vi "LoaderWithColor.vi"() -> ()   [LabVIEW 2019]
uses:
  <vilib>/Rock Robotics/WPI/ThirdParty/Phoenix-LabVIEW/Motor Controller/Controls/CTRE_Phoenix_MotorControl_ControlMode.ctl
  Robot Global Data.vi
  <vilib>/Rock Robotics/WPI/ThirdParty/Phoenix-LabVIEW/Motor Controller/Get/CTRE_Phoenix_MotorController_GetSelectedSensorData.vi
panel:
  out "Position":i32
  in  "counter":dbl
  in  "Output":dbl
  out "SEE?":bool
  out "intake":bool
  in  "error in":errorcluster
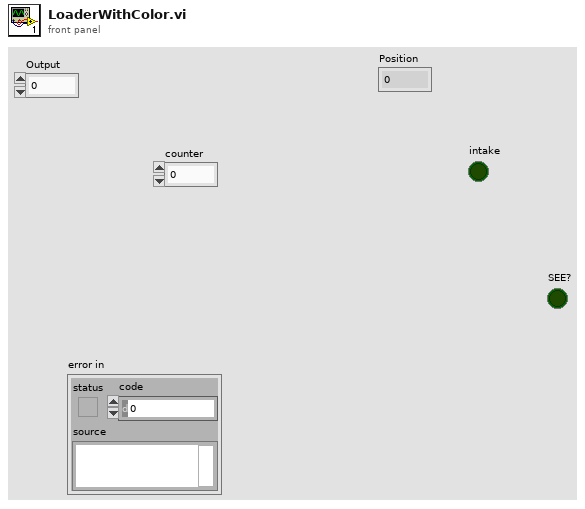
[diagram p1: front panel]
types:
  T1 = typedef "WPI_JoystickDevRef.ctl" = cluster{"Device":T2}
  T2 = typedef "WPI_JoystickDeviceEnum.ctl" = enum16{"USB 0", "USB 1", "USB 2", "USB 3", "USB 4", "USB 5"}
  T3 = typedef "WPI_MotorControlDeviceRef.ctl" = cluster{"DeviceStatus":errorcluster, "Type":T4, "PWM":cluster{"PWM Channel":T5, "DeadBand":T6}, "CAN":cluster{"Device Number":u8, "SetOutput VI Ref":variant, "GetOutput VI Ref":variant, "Enable VI Ref":variant, "Disable VI Ref":variant, "Data":variant}, "Invert":bool, "DIO PWM":cluster{"PWM \"Enable\" Channel":T5, "DIOChannel":T7, "PWM Rate":dbl}}
  T4 = typedef "WPI_MotorControlType.ctl" = enum16{"PWM", "CAN", "DIO PWM"}
  T5 = typedef "FPGA_DIOPWMChannel.ctl" = enum8{"PWM 0", "PWM 1", "PWM 2", "PWM 3", "PWM 4", "PWM 5", "PWM 6", "PWM 7", "PWM 8", "PWM 9", "PWM MXP 0", "PWM MXP 1", "PWM MXP 2", "PWM MXP 3", "PWM MXP 4", "PWM MXP 5", "PWM MXP 6", "PWM MXP 7", "PWM MXP 8", "PWM MXP 9", "Invalid"}
  T6 = typedef "WPI_PWMDeadband.ctl" = cluster{"Name":string, "maxPositivePwm":i32, "minPositivePwm":i32, "centerPwm":i32, "maxNegativePwm":i32, "minNegativePwm":i32, "angularRange":u16}
  T7 = typedef "FPGA_DIOChannel.ctl" = enum8{"DIO 0", "DIO 1", "DIO 2", "DIO 3", "DIO 4", "DIO 5", "DIO 6", "DIO 7", "DIO 8", "DIO 9", "DIO MXP 0", "DIO MXP 1", "DIO MXP 2", "DIO MXP 3", "DIO MXP 4", "DIO MXP 5", "DIO MXP 6", "DIO MXP 7", "DIO MXP 8", "DIO MXP 9", "DIO MXP 10", "DIO MXP 11", "DIO MXP 12", "DIO MXP 13", "DIO MXP 14", "DIO MXP 15", "SPI Port CS1", "SPI Port CS2", "SPI Port CS3", "SPI Port MISO", "SPI Port MOSI", "Invalid"}
  T8 = typedef "CTRE_Phoenix_MotorControl_ControlMode.ctl" = u16
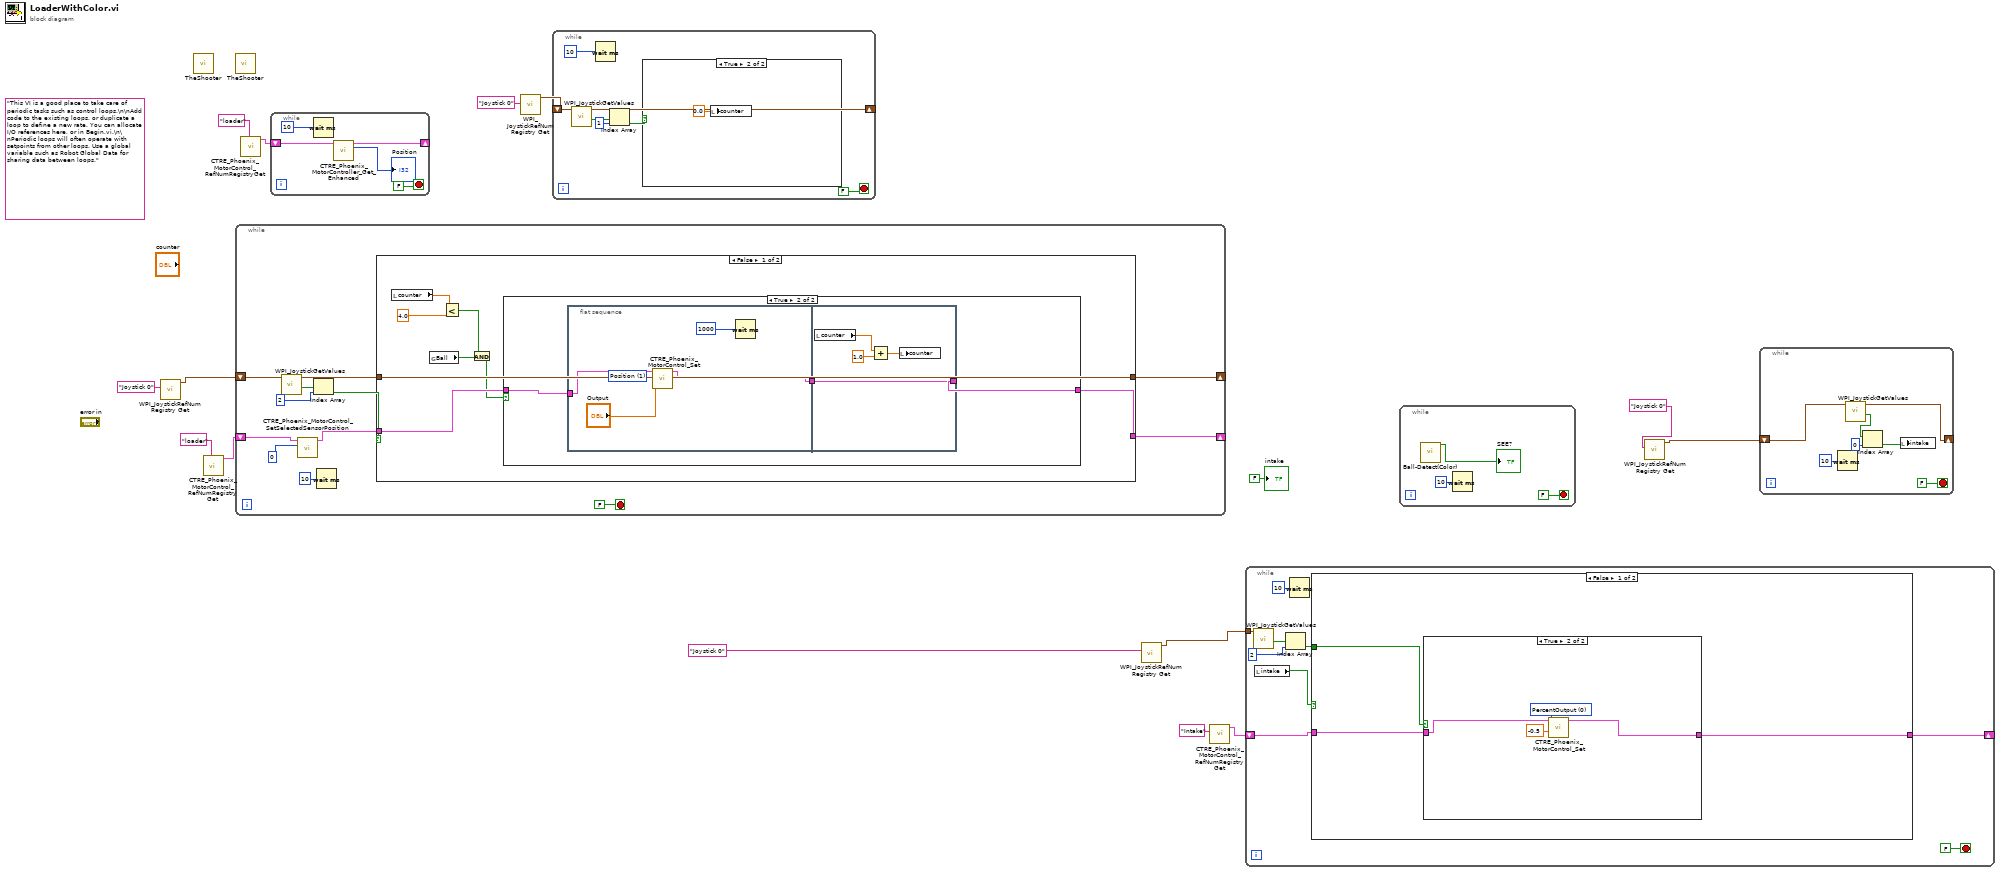
[diagram p0: block diagram]
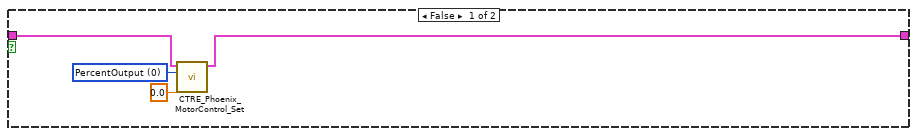
[diagram p3: hidden frame]
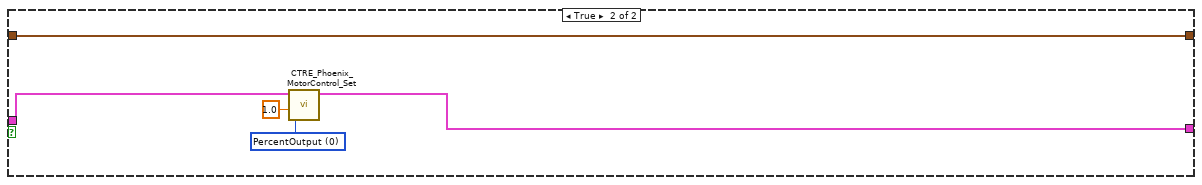
[diagram p4: hidden frame]
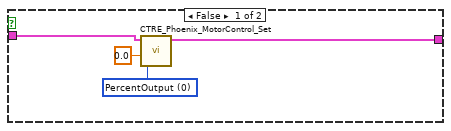
[diagram p5: hidden frame]
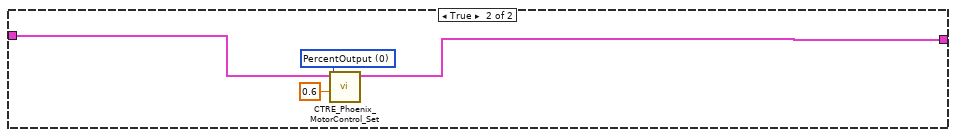
[diagram p6: hidden frame]
diagram:
  (unwired) "This VI is a good place to take care of periodic tasks such as control loops.\n\nAdd code to the existing loops, or duplicate a loop to define a new rate. You can allocate I/O references here, or in Begin.vi.\n\nPeriodic loops will often operate with setpoints from other loops. Use a global variable such as Robot Global Data for sharing data between loops."
  n1 = call <vilib>:"WPI_JoystickRefNum Registry Get.vi"("refnum name"="Joystick 0") -> ("JoystickDevRef"=w7:T1)  [unwired: 9 in, 1 out]
  n2 = call "TheShooter.vi"() -> ()  [unwired: 12 in]
  n3 = call <vilib>:"CTRE_Phoenix_MotorControl_RefNumRegistryGet.vi"("refnum name"="loader") -> ("PhoenixMotorControlDevRef"=w9:T3)  [unwired: 9 in, 1 out]
  n4 = call "TheShooter.vi"() -> ()  [unwired: 12 in]
  n5 = while {
    shift-right: [w25] -> _
    shift-left: w9 -> [w17]
    shift-right: [w21] -> _
    shift-left: w7 -> [w23]
    stop <- FALSE stop-if-true
    n6 = call <vilib>:"WPI_JoystickGetValues.vi"("JoystickDevRef"=w23) -> ("Buttons"=w24:bool[], "JoystickDevRef"=w22:T1)  [unwired: 6 in, 3 out]
    n7 = call <vilib>:"CTRE_Phoenix_MotorControl_SetSelectedSensorPosition.vi"("New Sensor Position"=0, "PhoenixMotorControlDevRef"=w17) -> ("PhoenixMotorControlDevRef"=w16:T3)  [unwired: 8 in, 1 out]
    n8 = Index Array(array=w24, index=2) -> (element=w20:bool)
    n9 = Wait (ms)(milliseconds to wait=u32 10) -> ()  [unwired: 1 out]
    n10 = case shown="False" w20 {
      tunnel: [w34 w53] -> w25
      tunnel: w16 -> [w35 w54]
      tunnel: w22 -> [w33 w52]
      tunnel: [w33 w52] -> w21
      frame False {
        n11 = local read "counter"() -> (w32:dbl)
        n12 = global read "Robot Global Data.vi" "Ball"() -> (w30:bool)
        n13 = Less?(x=w32, y=4.0) -> (x < y?=w28:bool)
        n14 = And(x=w28, y=w30) -> (x .and. y?=w29:bool)
        n15 = case shown="True" w29 {
          tunnel: w35 -> [w37 w40]
          tunnel: [w36 w42] -> w34
          frame False {
            w39 = T8 0 items=["PercentOutput"=0, "Position"=1, "Velocity"=2, "Current"=3, "Follower"=5, "MotionProfile"=6, "MotionMagic"=7, "MotionProfileArc"=10, "Disabled"=15] ("Control Mode")
            n16 = call <vilib>:"CTRE_Phoenix_MotorControl_Set.vi"("Output"=0.0, "Control Mode"=w39, "PhoenixMotorControlDevRef"=w37) -> ("PhoenixMotorControlDevRef"=w36:T3)  [unwired: 7 in, 1 out]
          }
          frame True {
            n17 = flat-sequence {
              tunnel: [w45] -> w41
              tunnel: w40 -> [w46]
              tunnel: [w51] -> w42
              tunnel: w41 -> [w51]
              frame #0 {
                w44 = T8 1 items=["PercentOutput"=0, "Position"=1, "Velocity"=2, "Current"=3, "Follower"=5, "MotionProfile"=6, "MotionMagic"=7, "MotionProfileArc"=10, "Disabled"=15] ("Control Mode")
                n18 = call <vilib>:"CTRE_Phoenix_MotorControl_Set.vi"("Output"="Output", "Control Mode"=w44, "PhoenixMotorControlDevRef"=w46) -> ("PhoenixMotorControlDevRef"=w45:T3)  [unwired: 7 in, 1 out]
                n19 = Wait (ms)(milliseconds to wait=u32 1000 ("millisecond timer value")) -> ()  [unwired: 1 out]
              }
              frame #1 {
                n20 = local read "counter"() -> (w49:dbl)
                n21 = Add(x=w49, y=1.0) -> (x+y=w50:dbl)
                n22 = local write "counter"(w50) -> ()
              }
            }
          }
        }
      }
      frame True {
        w55 = T8 0 items=["PercentOutput"=0, "Position"=1, "Velocity"=2, "Current"=3, "Follower"=5, "MotionProfile"=6, "MotionMagic"=7, "MotionProfileArc"=10, "Disabled"=15] ("Control Mode")
        n23 = call <vilib>:"CTRE_Phoenix_MotorControl_Set.vi"("Output"=1.0, "Control Mode"=w55, "PhoenixMotorControlDevRef"=w54) -> ("PhoenixMotorControlDevRef"=w53:T3)  [unwired: 7 in, 1 out]
      }
    }
  }
  n24 = call <vilib>:"CTRE_Phoenix_MotorControl_RefNumRegistryGet.vi"("refnum name"="loader") -> ("PhoenixMotorControlDevRef"=w1:T3)  [unwired: 9 in, 1 out]
  n25 = while {
    shift-right: [w60] -> _
    shift-left: w1 -> [w61]
    stop <- FALSE stop-if-true
    n26 = Wait (ms)(milliseconds to wait=u32 10 ("millisecond timer value")) -> ()  [unwired: 1 out]
    n27 = call-poly <vilib>:"CTRE_Phoenix_MotorController_Get_Enhanced.vi"("PhoenixMotorControlDevRef"=w61) -> ("PhoenixMotorControlDevRef"=w60:T3, "Position (Raw Sensor Units)"=→"Position":i32)  [unwired: 11 in, 2 out]
  }
  n28 = call <vilib>:"WPI_JoystickRefNum Registry Get.vi"("refnum name"="Joystick 0") -> ("JoystickDevRef"=w3:T1)  [unwired: 9 in, 1 out]
  n29 = while {
    shift-right: [w64] -> _
    shift-left: w3 -> [w66]
    stop <- FALSE stop-if-true
    n30 = call <vilib>:"WPI_JoystickGetValues.vi"("JoystickDevRef"=w66) -> ("Buttons"=w68:bool[], "JoystickDevRef"=w64:T1)  [unwired: 6 in, 3 out]
    n31 = Wait (ms)(milliseconds to wait=u32 10 ("millisecond timer value")) -> ()  [unwired: 1 out]
    n32 = Index Array(array=w68, index=1) -> (element=w65:bool)
    n33 = case shown="True" w65 {
      frame False {
      }
      frame True {
        n34 = local write "counter"(0.0 ("counter")) -> ()
      }
    }
  }
  n35 = call <vilib>:"WPI_JoystickRefNum Registry Get.vi"("refnum name"="Joystick 0") -> ("JoystickDevRef"=w5:T1)  [unwired: 9 in, 1 out]
  n36 = call <vilib>:"CTRE_Phoenix_MotorControl_RefNumRegistryGet.vi"("refnum name"="Intake") -> ("PhoenixMotorControlDevRef"=w12:T3)  [unwired: 9 in, 1 out]
  n37 = while {
    shift-right: [w75] -> _
    shift-left: w12 -> [w76]
    tunnel: w5 -> [w71]
    stop <- FALSE stop-if-true
    n38 = call <vilib>:"WPI_JoystickGetValues.vi"("JoystickDevRef"=w71) -> ("Buttons"=w72:bool[])  [unwired: 6 in, 4 out]
    n39 = local read "intake"() -> (w74:bool)
    n40 = Index Array(array=w72, index=2) -> (element=w70:bool)
    n41 = Wait (ms)(milliseconds to wait=u32 10) -> ()  [unwired: 1 out]
    n42 = case shown="False" w74 {
      tunnel: w76 -> [w81 w93]
      tunnel: [w80 w92] -> w75
      tunnel: w70 -> [w79 _]
      frame False {
        n43 = case shown="True" w79 {
          tunnel: w81 -> [w83 w87]
          tunnel: [w82 w86] -> w80
          frame False {
            w85 = T8 0 items=["PercentOutput"=0, "Position"=1, "Velocity"=2, "Current"=3, "Follower"=5, "MotionProfile"=6, "MotionMagic"=7, "MotionProfileArc"=10, "Disabled"=15] ("Control Mode")
            n44 = call <vilib>:"CTRE_Phoenix_MotorControl_Set.vi"("Output"=0.0, "Control Mode"=w85, "PhoenixMotorControlDevRef"=w83) -> ("PhoenixMotorControlDevRef"=w82:T3)  [unwired: 7 in, 1 out]
          }
          frame True {
            w89 = T8 0 items=["PercentOutput"=0, "Position"=1, "Velocity"=2, "Current"=3, "Follower"=5, "MotionProfile"=6, "MotionMagic"=7, "MotionProfileArc"=10, "Disabled"=15] ("Control Mode")
            n45 = call <vilib>:"CTRE_Phoenix_MotorControl_Set.vi"("Output"=-0.5, "Control Mode"=w89, "PhoenixMotorControlDevRef"=w87) -> ("PhoenixMotorControlDevRef"=w86:T3)  [unwired: 7 in, 1 out]
          }
        }
      }
      frame True {
        w91 = T8 0 items=["PercentOutput"=0, "Position"=1, "Velocity"=2, "Current"=3, "Follower"=5, "MotionProfile"=6, "MotionMagic"=7, "MotionProfileArc"=10, "Disabled"=15] ("Control Mode")
        n46 = call <vilib>:"CTRE_Phoenix_MotorControl_Set.vi"("Output"=0.6, "Control Mode"=w91, "PhoenixMotorControlDevRef"=w93) -> ("PhoenixMotorControlDevRef"=w92:T3)  [unwired: 7 in, 1 out]
      }
    }
  }
  n47 = while {
    stop <- FALSE stop-if-true
    n48 = call "Ball-Detect(Color).vi"() -> ("See"=→"SEE?":bool)  [unwired: 10 in]
    n49 = Wait (ms)(milliseconds to wait=u32 10) -> ()  [unwired: 1 out]
  }
  n50 = call <vilib>:"WPI_JoystickRefNum Registry Get.vi"("refnum name"="Joystick 0") -> ("JoystickDevRef"=w13:T1)  [unwired: 9 in, 1 out]
  n51 = while {
    shift-right: [w100] -> _
    shift-left: w13 -> [w101]
    stop <- FALSE stop-if-true
    n52 = Wait (ms)(milliseconds to wait=u32 10) -> ()  [unwired: 1 out]
    n53 = call <vilib>:"WPI_JoystickGetValues.vi"("JoystickDevRef"=w101) -> ("Buttons"=w99:bool[], "JoystickDevRef"=w100:T1)  [unwired: 6 in, 3 out]
    n54 = Index Array(array=w99, index=0) -> (element=w98:bool)
    n55 = local write "intake"(w98) -> ()
  }
  "intake" <- FALSE ("intake")
